vi "Counting blocks.vi"() -> ()   [LabVIEW 2015]
panel:
  in  "stop":bool
  out "block count":i32
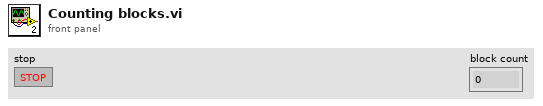
[diagram p1: front panel]
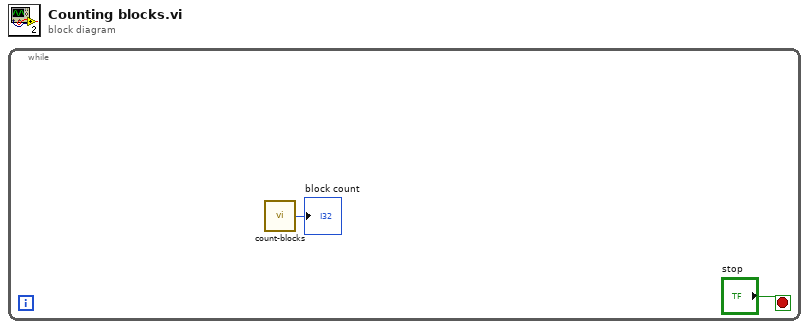
[diagram p0: block diagram]
diagram:
  n1 = while {
    stop <- "stop" stop-if-true
    n2 = call "count-blocks.vi"() -> ("block count"=→"block count":i32)
  }
